vi "Close Connection.vi"(8 "error in (no error)":errorcluster, 11 "REST Client in":refnum<class "REST Client.lvclass">) -> (0 "error out":errorcluster)   [LabVIEW 2021, in "G5 Regatron Custom Device Engine.lvlib"]
uses:
  G5 Regatron Custom Device Engine.lvlib
  <vilib>/addons/_JKI.lib/REST Client/classes/REST Client/REST Client.lvclass
  Shared/Regatron.G5.Rest.lvlib
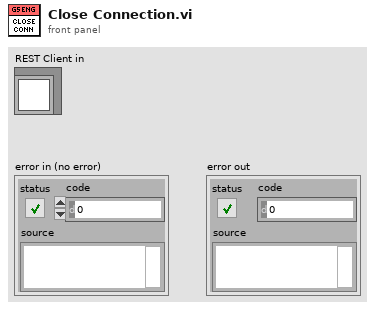
[diagram p1: front panel]
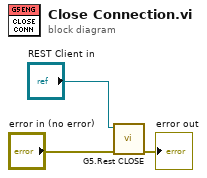
[diagram p0: block diagram]
diagram:
  n1 = call "G5.Rest CLOSE.vi"("Fehler (Eingang, kein Fehler)"="error in (no error)", "G5 WEB API"="REST Client in") -> ("error out"=→"error out":errorcluster)  [unwired: 9 in]
